vi "CreateLimitExpression.vi"(8 "error in":errorcluster, 9 "HigherBound":string, 10 "LowerBound":string, 11 "ComparisonType":T1) -> (0 "error out":errorcluster, 3 "LimitExpression":string)   [LabVIEW 2021, in "ProligentXMLGenerator.lvlib" / "RangeMeasureLimit.lvclass"]
uses:
  RangeMeasureLimit.lvclass
  RangeMeasureLimit.lvclass/RangeMeasureLimit.ctl
  ComparisonType.ctl
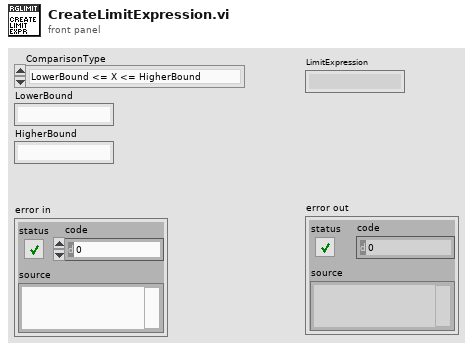
[diagram p1: front panel]
types:
  T1 = typedef "ProligentXMLGenerator.lvlib/RangeMeasureLimit.lvclass/ComparisonType.ctl" = enum16{"LowerBound <= X <= HigherBound", "LowerBound < X <= HigherBound", "LowerBound <= X < HigherBound", "LowerBound < X < HigherBound", "LowerBound <= X", "LowerBound < X", "X <= HigherBound", "X < HigherBound", "X == HigherBound", "X != HigherBound", "X <= LowerBound OR HigherBound <= X", "X < LowerBound OR HigherBound <= X", "X <= LowerBound OR HigherBound < X", "X < LowerBound OR HigherBound < X"}
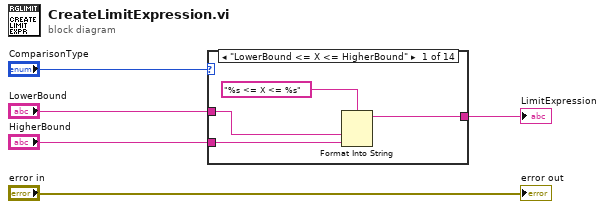
[diagram p0: block diagram]
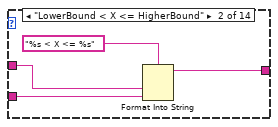
[diagram p2: hidden frame]
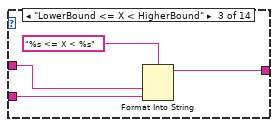
[diagram p3: hidden frame]
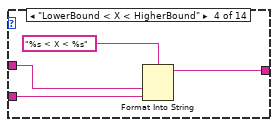
[diagram p4: hidden frame]
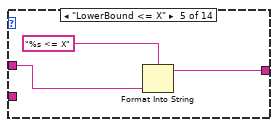
[diagram p5: hidden frame]
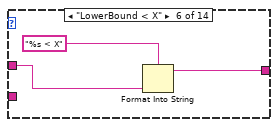
[diagram p6: hidden frame]
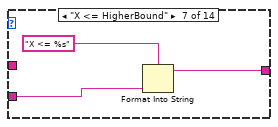
[diagram p7: hidden frame]
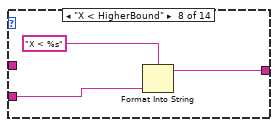
[diagram p8: hidden frame]
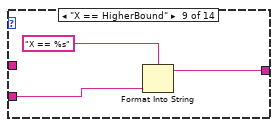
[diagram p9: hidden frame]
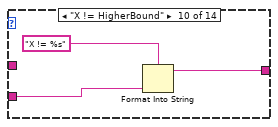
[diagram p10: hidden frame]
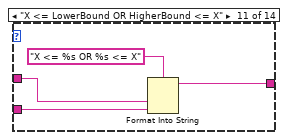
[diagram p11: hidden frame]
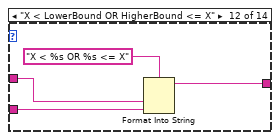
[diagram p12: hidden frame]
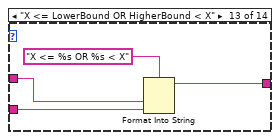
[diagram p13: hidden frame]
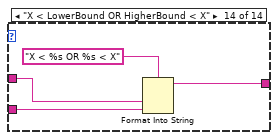
[diagram p14: hidden frame]
diagram:
  n1 = case shown="\"LowerBound <= X <= HigherBound\"" "ComparisonType" {
    tunnel: "HigherBound" -> [w8 w12 w16 w20 _ _ w30 w33 w36 w39 w42 w46 w50 w54]
    tunnel: "LowerBound" -> [w9 w13 w17 w21 w24 w27 _ _ _ _ w41 w45 w49 w53]
    tunnel: [w7 w11 w15 w19 w23 w26 w29 w32 w35 w38 w43 w47 w51 w55] -> w5
    frame "LowerBound <= X <= HigherBound" {
      n2 = Format Into String(format string="%s <= X <= %s", w9, w8) -> (resulting string=w7:string)  [unwired: 2 in, 1 out]
    }
    frame "LowerBound < X <= HigherBound" {
      n3 = Format Into String(format string="%s < X <= %s", w13, w12) -> (resulting string=w11:string)  [unwired: 2 in, 1 out]
    }
    frame "LowerBound <= X < HigherBound" {
      n4 = Format Into String(format string="%s <= X < %s", w17, w16) -> (resulting string=w15:string)  [unwired: 2 in, 1 out]
    }
    frame "LowerBound < X < HigherBound" {
      n5 = Format Into String(format string="%s < X < %s", w21, w20) -> (resulting string=w19:string)  [unwired: 2 in, 1 out]
    }
    frame "LowerBound <= X" {
      n6 = Format Into String(format string="%s <= X", w24) -> (resulting string=w23:string)  [unwired: 2 in, 1 out]
    }
    frame "LowerBound < X" {
      n7 = Format Into String(format string="%s < X", w27) -> (resulting string=w26:string)  [unwired: 2 in, 1 out]
    }
    frame "X <= HigherBound" {
      n8 = Format Into String(format string="X <= %s", w30) -> (resulting string=w29:string)  [unwired: 2 in, 1 out]
    }
    frame "X < HigherBound" {
      n9 = Format Into String(format string="X < %s", w33) -> (resulting string=w32:string)  [unwired: 2 in, 1 out]
    }
    frame "X == HigherBound" {
      n10 = Format Into String(format string="X == %s", w36) -> (resulting string=w35:string)  [unwired: 2 in, 1 out]
    }
    frame "X != HigherBound" {
      n11 = Format Into String(format string="X != %s", w39) -> (resulting string=w38:string)  [unwired: 2 in, 1 out]
    }
    frame "X <= LowerBound OR HigherBound <= X" {
      n12 = Format Into String(format string="X <= %s OR %s <= X", w41, w42) -> (resulting string=w43:string)  [unwired: 2 in, 1 out]
    }
    frame "X < LowerBound OR HigherBound <= X" {
      n13 = Format Into String(format string="X < %s OR %s <= X", w45, w46) -> (resulting string=w47:string)  [unwired: 2 in, 1 out]
    }
    frame "X <= LowerBound OR HigherBound < X" {
      n14 = Format Into String(format string="X <= %s OR %s < X", w49, w50) -> (resulting string=w51:string)  [unwired: 2 in, 1 out]
    }
    frame "X < LowerBound OR HigherBound < X" {
      n15 = Format Into String(format string="X < %s OR %s < X", w53, w54) -> (resulting string=w55:string)  [unwired: 2 in, 1 out]
    }
  }
  "LimitExpression" <- w5
  "error out" <- "error in"
